vi "UNITTEST-JSON-RPC-Flatten.vi"(8 "error in (no error)":errorcluster) -> (0 "error out":errorcluster)   [LabVIEW 2019]
uses:
  <vilib>/numeric/Random Number (Range) DBL.vi
  e2ac90a9-f3dc-4cb2-8134-752160e7079c.vi
  f7cbbd81-eb58-4d71-bada-c91a7ecadc85.vi
  a1118f79-2200-4914-8c15-bf3ed6399d3b.vi
  f401dca3-f631-40e3-af1b-75a836bd8272.vi
  <vilib>/JDP Science/JSONtext/Make JSON Array.vi
  f7cbbd81-eb58-4d71-bada-c91a7ecadc85.vi/acbb5ffe-10a4-453b-89eb-0f66d56dfa07.vi
  f401dca3-f631-40e3-af1b-75a836bd8272.vi/e7582be5-ae4a-484e-84a1-3d69075d4ca4.vi
  <vilib>/JDP Science/JSONtext/Variant to JSON Text.vi
  <vilib>/JDP Science/JSONtext/support/Format JSON Array Text.vi
  <vilib>/JDP Science/JSONtext/JSON text to Variant.vi
  <vilib>/addons/_JKI Toolkits/Caraya/classes/Assert/Assert Equal Value_Variant.vi
  <vilib>/addons/_JKI Toolkits/Caraya/classes/Assert/Assert Not Error.vi
  <vilib>/JDP Science/JSONtext/LVClass Serializer/JSONtext LVClass Serializer.lvclass
  JSON-RPC/JSON-RPC.lvclass
  <vilib>/addons/_JKI Toolkits/Caraya/classes/Assert/Assert.lvclass
  <vilib>/addons/_JKI Toolkits/Caraya/classes/Test/Test.lvclass
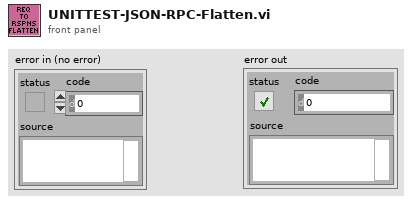
[diagram p1: front panel]
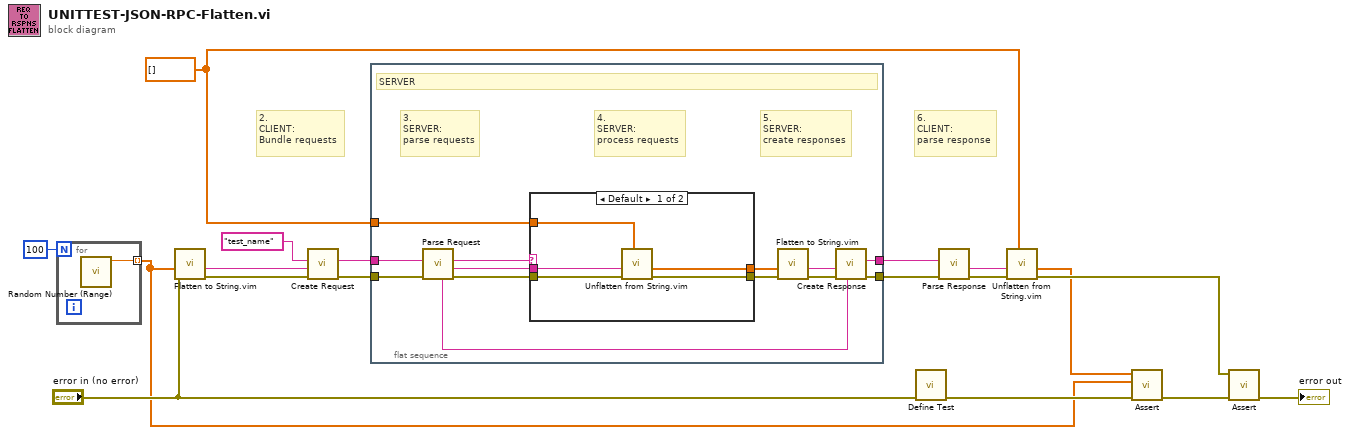
[diagram p0: block diagram]
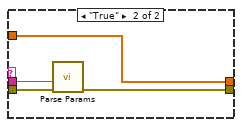
[diagram p2: hidden frame]
diagram:
  w6 = dbl[] []
  # "6.\nCLIENT:\nparse response"
  # "2.\nCLIENT:\nBundle requests"
  n1 = for {
    N: 100 -> [_]
    tunnel: [w19] -> w4 mode=indexing
    n2 = call-poly <vilib>:"Random Number (Range).vi"() -> ("number"=w19:dbl)  [unwired: 11 in]
  }
  n3 = call "Flatten to String.vim"("error in (no error)"="error in (no error)", "Data in"=w4) -> ("error out"=w9:errorcluster, "<JSON>"=w3:string)  [unwired: 8 in]
  n4 = call "Create Request.vi"("error in (no error)"=w9, "params"=w3, "method"="test_name") -> ("error out"=w17:errorcluster, "<JSON> Requests"=w18:string)  [unwired: 5 in, 2 out]
  n5 = flat-sequence {
    tunnel: w18 -> [w32]
    tunnel: w17 -> [w28]
    tunnel: [w27] -> w16
    tunnel: [w26] -> w15
    tunnel: w6 -> [w25]
    frame #0 {
      # "3.\nSERVER:\nparse requests"
      # "4.\nSERVER:\nprocess requests"
      # "5.\nSERVER:\ncreate responses"
      # "SERVER"
      n6 = call "Parse Request.vi"("error in (no error)"=w28, "<JSON> Requests"=w32) -> ("error out"=w29:errorcluster, "Params"=w30:string, "Methods"=w31:string, "IDs"=w22:string)  [unwired: 5 in, 1 out]
      n7 = case shown="Default" w31 {
        tunnel: w30 -> [w34 w41]
        tunnel: w29 -> [w37 w40]
        tunnel: [w36 w39] -> w23
        tunnel: w25 -> [w35 w38]
        tunnel: [w33 w38] -> w21
        frame Default {
          n8 = call "Unflatten from String.vim"("type"=w35, "error in (no error)"=w37, "<JSON>"=w34) -> ("error out"=w36:errorcluster, "Data out"=w33:dbl[])  [unwired: 7 in]
        }
        frame "True" {
          n9 = call "Parse Params.vi"("error in (no error)"=w40, "{JSON} Params"=w41) -> ("error out"=w39:errorcluster)  [unwired: 6 in, 3 out]
        }
      }
      n10 = call "Flatten to String.vim"("error in (no error)"=w23, "Data in"=w21) -> ("error out"=w24:errorcluster, "<JSON>"=w20:string)  [unwired: 8 in]
      n11 = call "Create Response.vi"("id"=w22, "error in (no error)"=w24, "result"=w20) -> ("error out"=w26:errorcluster, "<JSON> Response"=w27:string)  [unwired: 6 in, 1 out]
    }
  }
  n12 = call <vilib>:"Define Test.vi"("error in (no error)"="error in (no error)") -> ("error out"=w11:errorcluster)  [unwired: 9 in, 1 out]
  n13 = call "Parse Response.vi"("error in (no error)"=w15, "<JSON> Response"=w16) -> ("error out"=w8:errorcluster, "results"=w1:string)  [unwired: 5 in, 3 out]
  n14 = call "Unflatten from String.vim"("type"=w6, "error in (no error)"=w8, "<JSON>"=w1) -> ("error out"=w7:errorcluster, "Data out"=w2:dbl[])  [unwired: 7 in]
  n15 = call-poly <vilib>:"Assert.vi"("error in (no error)"=w11, "Y"=w4, "X"=w2) -> ("error out"=w14:errorcluster)  [unwired: 7 in, 1 out]
  n16 = call-poly <vilib>:"Assert.vi"("error in (no error)"=w14, "Not Error?"=w7) -> ("error out"=→"error out":errorcluster)  [unwired: 8 in, 1 out]
